vi "Check Generation Running State.vi"(8 "error in (no error)":errorcluster, 11 "Panel State Data In":T1={"FGEN Resource"="", "DAQmx Tasks Session"={"DO Task"="", "Ctr0 Task"=""}, "Scope Resource"="", "FGEN Enabled?"=FALSE, "DAQ Enabled?"=FALSE, "Scope Enabled?"=FALSE, "Max Total FGEN Wfm Duration (s)"=0.0, "FGEN-DAQ Routing"={"FGEN Start Trigger"="", "DAQ Trig Line"=""}, "Scope Recording Settings"={"Number of Records"=0, "Channels Per Record"=1, "Plot Names"=[], "Fetch Timeout"=0.0, "Channel List"=""}} {"Scope Recording Settings"."Fetch Timeout" format="%.2f"}) -> (0 "error out":errorcluster, 2 "Is Done?":bool, 3 "Panel State Data Out":T1={"FGEN Resource"="", "DAQmx Tasks Session"={"DO Task"="", "Ctr0 Task"=""}, "Scope Resource"="", "FGEN Enabled?"=FALSE, "DAQ Enabled?"=FALSE, "Scope Enabled?"=FALSE, "Max Total FGEN Wfm Duration (s)"=0.0, "FGEN-DAQ Routing"={"FGEN Start Trigger"="", "DAQ Trig Line"=""}, "Scope Recording Settings"={"Number of Records"=0, "Channels Per Record"=1, "Plot Names"=[], "Fetch Timeout"=0.0, "Channel List"=""}} {"Scope Recording Settings"."Fetch Timeout" format="%.2f"})   [LabVIEW 2025]
uses:
  Typedef/Test Panel State Data.ctl
  Typedef/Scope Recording Settings.ctl
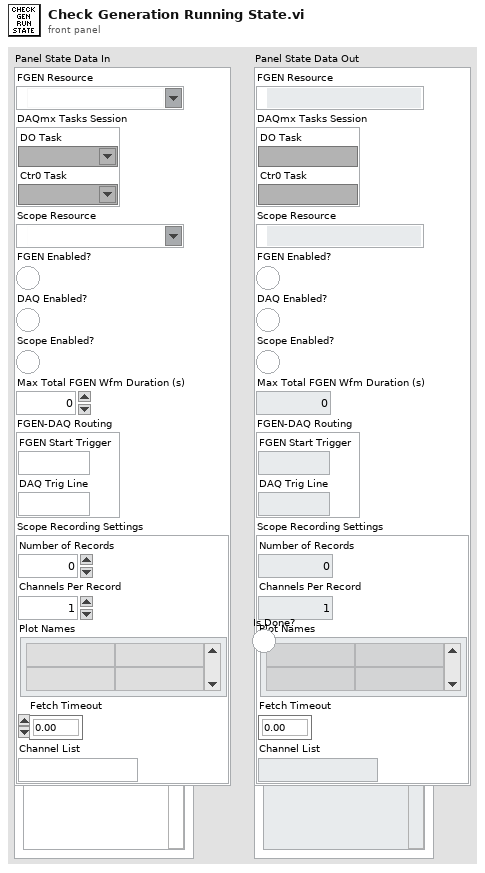
[diagram p1: front panel]
types:
  T1 = typedef "Test Panel State Data.ctl" = cluster{"FGEN Resource":refnum<k15>, "DAQmx Tasks Session":cluster{"DO Task":refnum<k21>, "Ctr0 Task":refnum<k21>}, "Scope Resource":refnum<k15>, "FGEN Enabled?":bool, "DAQ Enabled?":bool, "Scope Enabled?":bool, "Max Total FGEN Wfm Duration (s)":dbl, "FGEN-DAQ Routing":cluster{"FGEN Start Trigger":string, "DAQ Trig Line":string}, "Scope Recording Settings":T2}
  T2 = typedef "Scope Recording Settings.ctl" = cluster{"Number of Records":i32, "Channels Per Record":i32, "Plot Names":string[][], "Fetch Timeout":dbl, "Channel List":string}
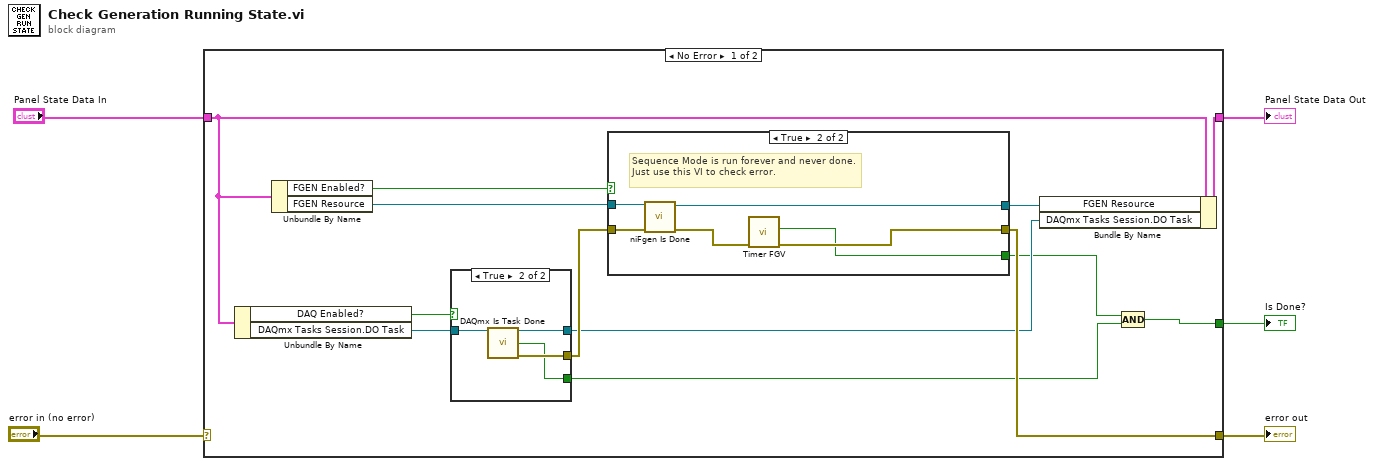
[diagram p0: block diagram]
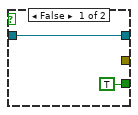
[diagram p2: hidden frame]
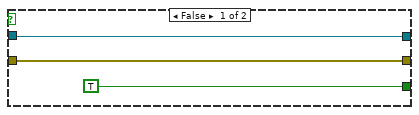
[diagram p3: hidden frame]
diagram:
  n1 = case shown="No Error" "error in (no error)" {
    selector: "error in (no error)" -> [_ w35]
    tunnel: "Panel State Data In" -> [w14 w34]
    tunnel: [w12 w35] -> w3
    tunnel: [w11 w34] -> w4
    tunnel: [w6 _] -> w1
    frame No Error {
      n2 = Unbundle By Name(w14) -> ("DAQ Enabled?"=w15:bool, "DAQmx Tasks Session.DO Task"=w16:refnum<k21>)
      n3 = Unbundle By Name(w14) -> ("FGEN Enabled?"=w18:bool, "FGEN Resource"=w17:refnum<k15>)
      n4 = case shown="True" w15 {
        tunnel: w16 -> [w20 w24]
        tunnel: [_ w23] -> w13
        tunnel: [w20 w22] -> w9
        tunnel: [TRUE ("task done?") w21] -> w7
        frame False {
        }
        frame True {
          n5 = call <vilib>:"DAQmx Is Task Done.vi"("task/channels in"=w24) -> ("task out"=w22:refnum<k21>, "task done?"=w21:bool, "error out"=w23:errorcluster)  [unwired: 12 in]
        }
      }
      n6 = case shown="True" w18 {
        tunnel: w17 -> [w26 w33]
        tunnel: [w27 w29] -> w12
        tunnel: w13 -> [w27 w31]
        tunnel: [w26 w30] -> w10
        tunnel: [TRUE ("Done") w28] -> w8
        frame False {
        }
        frame True {
          # "Sequence Mode is run forever and never done. Just use this VI to check error."
          n7 = call <instrlib>:"niFgen Is Done.vi"("error in (no error)"=w31, "Instrument Handle"=w33) -> ("error out"=w32:errorcluster, "Instrument Handle Out"=w30:refnum<k15>)  [unwired: 7 in, 1 out]
          n8 = call "Timer FGV.vi"("error in (no error)"=w32) -> ("error out"=w29:errorcluster, "Time Elapsed?"=w28:bool)  [unwired: 7 in, 2 out]
        }
      }
      n9 = Bundle By Name(cluster=w14, "FGEN Resource"=w10, "DAQmx Tasks Session.DO Task"=w9) -> (w11:T1)
      n10 = Compound Arithmetic op=AND(w8, w7) -> (w6:bool)
    }
    frame Error {
    }
  }
  "error out" <- w3
  "Panel State Data Out" <- w4
  "Is Done?" <- w1
